vi "RangeCheck.vi"(0 "AcPwrBase in":refnum<class "AcPwrBase.lvclass">, 1 "ValueNames":string[](array[string]), 2 "Phase":i32, 3 "error in (no error)":errorcluster) -> (7 "AcPwrBase out":refnum<class "AcPwrBase.lvclass">, 10 "error out":errorcluster)   [LabVIEW 2014, in "AcPwrPlugins.lvlib" / "AcPwrBase.lvclass"]
uses:
  AcPwrBase.lvclass
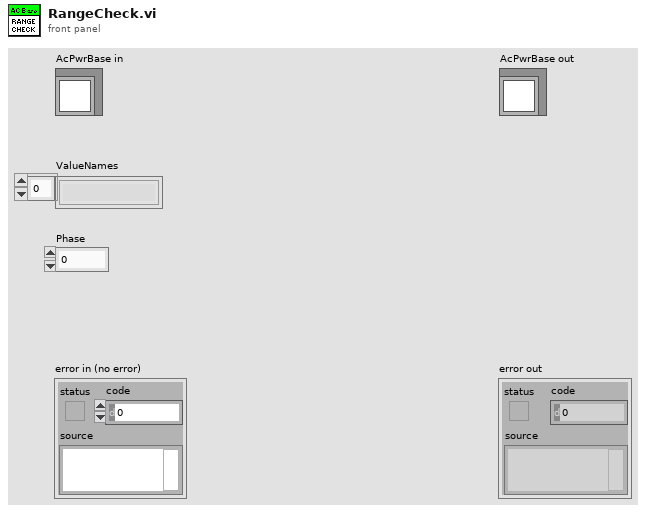
[diagram p1: front panel]
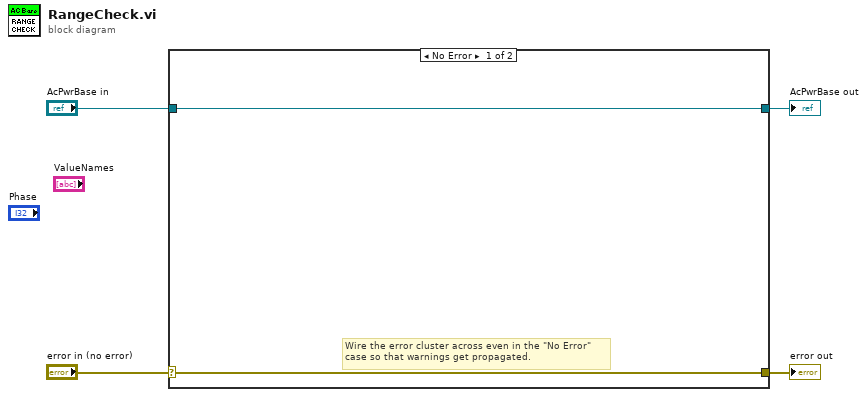
[diagram p0: block diagram]
diagram:
  n1 = case shown="No Error" "error in (no error)" {
    selector: "error in (no error)" -> [w5 w8]
    tunnel: [w5 w8] -> w3
    tunnel: [w6 w7] -> w1
    tunnel: "AcPwrBase in" -> [w6 w7]
    frame No Error {
      # "Wire the error cluster across even in the \"No Error\"\ncase so that warnings get propagated."
    }
    frame Error {
    }
  }
  "error out" <- w3
  "AcPwrBase out" <- w1
